vi "pyvigmentize.vi"(0 "Text Field Destination":refnum<vi>, 1 "style name (material)":string="material", 7 "String":string) -> ()   [LabVIEW 2025]
uses:
  Text Style Definition.ctl
  <vilib>/regexp/Match Regular Expression.xnode
panel:
  out "error out":errorcluster
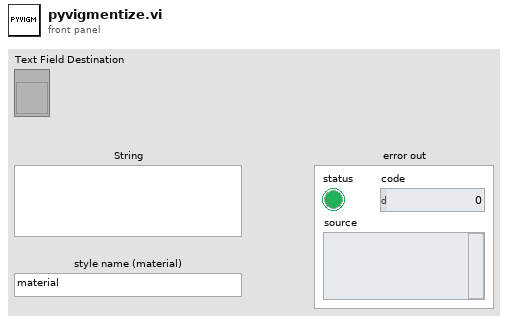
[diagram p1: front panel]
types:
  T1 = cluster{"Python version":string[], "Python version":string[]}
  T2 = typedef "Text Style Definition.ctl" = cluster{"FG color":u32, "bold":bool, "italic":bool, "underline":bool, "roman":bool, "sans":bool, "mono":bool, "strikethrough":bool, "BG color":u32}
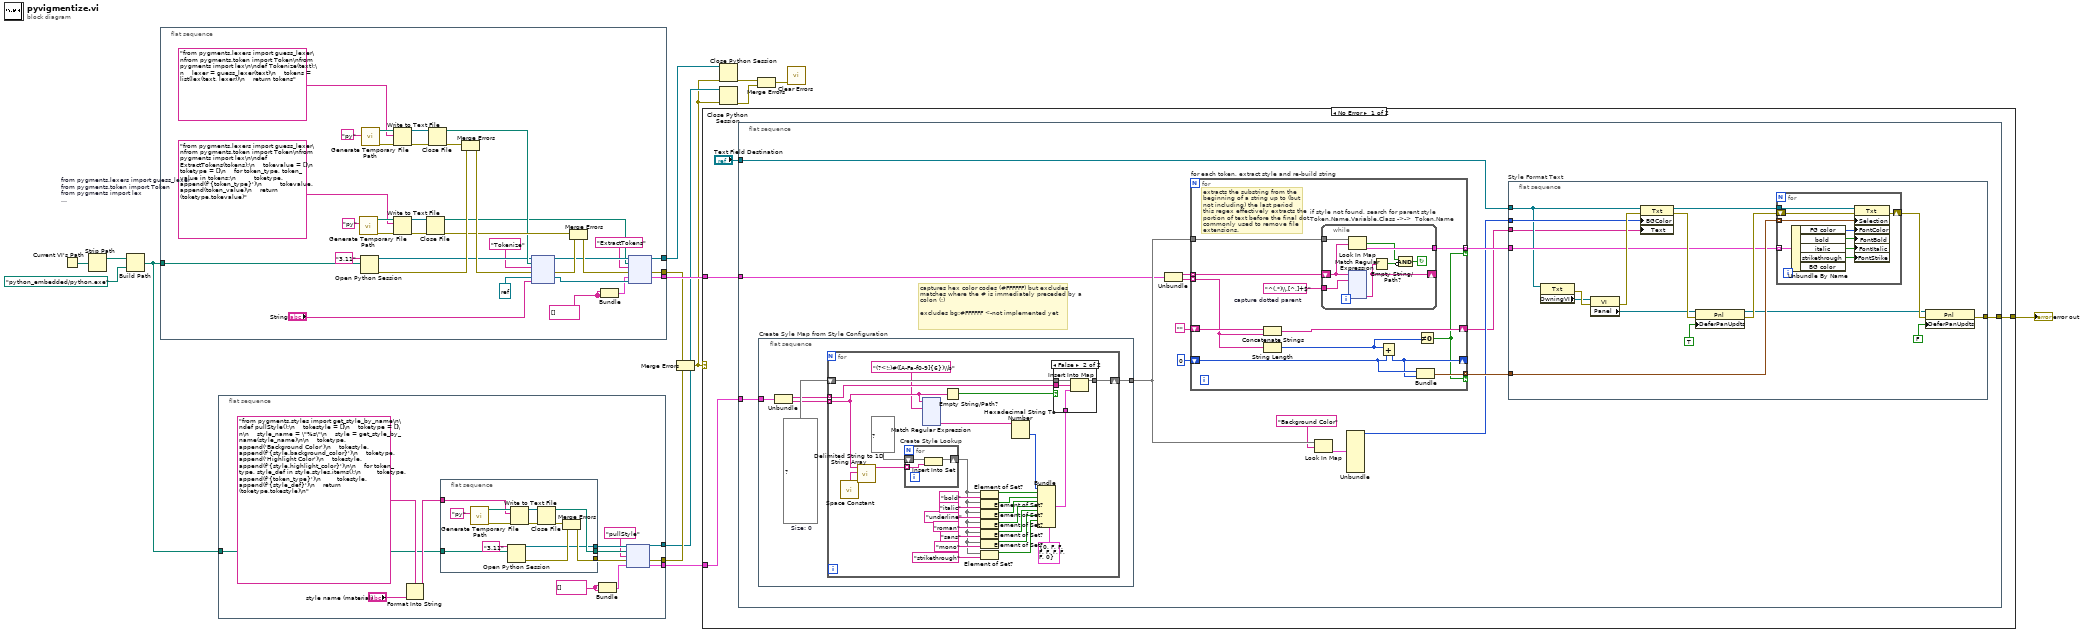
[diagram p0: block diagram]
diagram:
  n1 = Current VI's Path() -> (path=w4:path)
  n2 = Strip Path(path=w4) -> (stripped path=w2:path)  [unwired: 1 out]
  n3 = Build Path(base path=w2, name or relative path=path "python_embedded/python.exe" ("python path")) -> (appended path=w1:path)
  n4 = flat-sequence {
    tunnel: [w41] -> w12
    tunnel: [w22] -> w14
    tunnel: w1 -> [w17]
    tunnel: [w16] -> w10
    frame #0 {
      w18 = "from pygments.lexers import guess_lexer\nfrom pygments.token import Token\nfrom pygments import lex\n\ndef ExtractTokens(tokens):\n    tokevalue = []\n    toketype = []\n    for token_type, token_value in tokens:\n         toketype.append(f'{token_type}')\n         tokevalue.append(token_value)\n    return (toketype,tokevalue)"  # from pygments.lexers import guess_lexer from pygments.token import Token from pygments import lex  def ExtractTokens(tokens):     tokevalue = []     toketype = []     for token_type, token_value in tokens:          toketype.append(f'{token_type}')          tokevalue.append(token_value)     return (toketype,tokevalue)
      w19 = string[] [] ("Python version")
      n5 = call <vilib>:"Generate Temporary File Path.vi"("Temporary File Extension (tmp)"="py") -> ("error out"=w46:errorcluster, "Unique Temporary File Path"=w34:path)  [unwired: 9 in]
      n6 = Open Python Session(python version="3.11" ("Python version"), python path=w17) -> (session out=w29:refnum<k35>, error out=w44:errorcluster)  [unwired: 1 in]
      n7 = call <vilib>:"Generate Temporary File Path.vi"("Temporary File Extension (tmp)"="py") -> ("error out"=w47:errorcluster, "Unique Temporary File Path"=w35:path)  [unwired: 9 in]
      n8 = Write to Text File(file (use dialog)=w35, text="from pygments.lexers import guess_lexer\nfrom pygments.token import Token\nfrom pygments import lex\n\ndef Tokenize(text):\n    lexer = guess_lexer(text)\n    tokens = list(lex(text, lexer))\n    return tokens", error in=w47) -> (refnum out=w38:refnum<file>, error out=w48:errorcluster)  [unwired: 1 in, 1 out]
      n9 = Write to Text File(file (use dialog)=w34, text=w18, error in=w46) -> (refnum out=w32:refnum<file>, error out=w45:errorcluster)  [unwired: 1 in, 1 out]
      n10 = Close File(refnum=w32, error in=w45) -> (path=w26:path, error out=w42:errorcluster)
      n11 = Close File(refnum=w38, error in=w48) -> (path=w30:path, error out=w49:errorcluster)
      n12 = Merge Errors(w49, w44) -> (w43:errorcluster)
      n13 = node(w29, w30, "Tokenize" ("function name"), w43, refnum<k38> refnum ("Python Object Refnum"), "String") -> (w31:refnum<k35>, w40:errorcluster, w24:refnum<k38>)  [unwired: 1 in, 2 out]
      n14 = Merge Errors(w42, w40) -> (w39:errorcluster)
      n15 = Bundle("Python version"=w19, "Python version"=w19) -> (w21:T1)  [unwired: 1 in]
      n16 = node(w31, w26, "ExtractTokens" ("function name"), w39, w21, w24) -> (w16:refnum<k35>, w41:errorcluster, w22:T1)  [unwired: 1 in, 2 out]
    }
  }
  n17 = flat-sequence {
    tunnel: [w57] -> w15
    tunnel: [w52] -> w11
    tunnel: w1 -> [w51]
    tunnel: [w50] -> w9
    frame #0 {
      w56 = string[] [] ("Python version")
      n18 = Format Into String(format string="from pygments.styles import get_style_by_name\n\ndef pullStyle():\n    tokestyle = []\n    toketype = []\n\n    style_name = \"%s\"\n    style = get_style_by_name(style_name)\n\n    toketype.append('Background Color')\n    tokestyle.append(f'{style.background_color}')\n    toketype.append('Highlight Color')\n    tokestyle.append(f'{style.highlight_color}')\n\n    for token_type, style_def in style.styles.items():\n        toketype.append(f'{token_type}')\n        tokestyle.append(f'{style_def}')\n    return (toketype,tokestyle)\n" ("text"), "style name (material)") -> (resulting string=w54:string)  [unwired: 2 in, 1 out]
      n19 = flat-sequence {
        tunnel: [w66] -> w61
        tunnel: [w65] -> w60
        tunnel: [w71] -> w62
        tunnel: w54 -> [w64]
        tunnel: w51 -> [w63]
        frame #0 {
          n20 = call <vilib>:"Generate Temporary File Path.vi"("Temporary File Extension (tmp)"="py") -> ("error out"=w75:errorcluster, "Unique Temporary File Path"=w68:path)  [unwired: 9 in]
          n21 = Open Python Session(python version="3.11" ("Python version"), python path=w63) -> (session out=w65:refnum<k35>, error out=w72:errorcluster)  [unwired: 1 in]
          n22 = Write to Text File(file (use dialog)=w68, text=w64, error in=w75) -> (refnum out=w67:refnum<file>, error out=w74:errorcluster)  [unwired: 1 in, 1 out]
          n23 = Close File(refnum=w67, error in=w74) -> (path=w66:path, error out=w73:errorcluster)
          n24 = Merge Errors(w73, w72) -> (w71:errorcluster)
        }
      }
      n25 = Bundle("Python version"=w56, "Python version"=w56) -> (w58:T1)  [unwired: 1 in]
      n26 = node(w60, w61, "pullStyle" ("function name"), w62, w58) -> (w50:refnum<k35>, w52:errorcluster, w57:T1)  [unwired: 2 out]
    }
  }
  n27 = Merge Errors(w12, w11) -> (w8:errorcluster)
  n28 = case shown="No Error" w8 {
    selector: w8 -> [_ w420]
    tunnel: w15 -> [w79 _]
    tunnel: w14 -> [w78 _]
    tunnel: [w76 w420] -> w13
    frame No Error {
      n29 = flat-sequence {
        tunnel: w79 -> [w91]
        tunnel: w78 -> [w86]
        tunnel: "Text Field Destination" -> [w84]
        tunnel: [w81] -> w76
        frame #0 {
          # "captures hex color codes (#FFFFFF) but excludes matches where the # is immediately preceded by a colon (:)\n\nexcludes bg:#FFFFFF <-not implemented yet"
          n30 = flat-sequence "Create Syle Map from Style Configuration" {
            tunnel: [w125] -> w89
            tunnel: w91 -> [w123]
            frame #0 {
              w124 = map{string, T2} {}  # Size: 0
              n31 = Unbundle(w123) -> ("Python version"=w122:string[], "Python version"=w121:string[])
              n32 = for {
                tunnel: w122 -> [w134] mode=indexing
                shift-right: [w153] -> w125
                shift-left: w124 -> [w152]
                tunnel: w121 -> [w131] mode=indexing
                n33 = call <vilib>:"Space Constant.vi"() -> ("String"=w151:string)
                n34 = call <vilib>:"Delimited String to 1D String Array.vi"("delimiter"=w151, "delimited string"=w131) -> ("string array"=w132:string[])  [unwired: 9 in]
                n35 = for "Create Style Lookup" {
                  tunnel: w132 -> [w279] mode=indexing
                  shift-right: [w278] -> w127
                  shift-left: set{string} {} ("set") -> [w280]
                  n36 = Insert Into Set(10:w279, 11:w280) -> (3:w278:set{string})  [unwired: 1 out]
                }
                n37 = xnode "Match Regular Expression"("input string"=w131, "regular expression"="(?<!:)#([A-Fa-f0-9]{6})\\b") -> ("submatch 1"=w129:string)  [unwired: 4 in, 5 out]
                n38 = Empty String/Path?(string/path=w131) -> (empty?=w133:bool)
                n39 = Element of Set?(10:"bold", 11:w127) -> (3:w143:bool)
                n40 = Element of Set?(10:"italic", 11:w127) -> (3:w142:bool)
                n41 = Element of Set?(10:"underline", 11:w127) -> (3:w141:bool)
                n42 = Element of Set?(10:"roman", 11:w127) -> (3:w137:bool)
                n43 = Element of Set?(10:"sans", 11:w127) -> (3:w140:bool)
                n44 = Element of Set?(10:"mono", 11:w127) -> (3:w139:bool)
                n45 = Element of Set?(10:"strikethrough", 11:w127) -> (3:w126:bool)
                n46 = Hexadecimal String To Number(string=w129) -> (number=w150:u32)  [unwired: 2 in, 1 out]
                n47 = Bundle(cluster=T2 {"FG color"=0, "bold"=FALSE, "italic"=FALSE, "underline"=FALSE, "roman"=FALSE, "sans"=FALSE, "mono"=FALSE, "strikethrough"=FALSE, "BG color"=0}, "FG color"=w150, "bold"=w143, "italic"=w142, "underline"=w141, "roman"=w137, "sans"=w140, "mono"=w139, "strikethrough"=w126) -> (w138:T2)  [unwired: 1 in]
                n48 = case shown="False" w133 {
                  tunnel: w134 -> [_ w277]
                  tunnel: [w273 w276] -> w153
                  tunnel: w152 -> [w273 w275]
                  tunnel: w138 -> [_ w274]
                  frame True {
                  }
                  frame False {
                    n49 = Insert Into Map(map in=w275, key=w277, value=w274) -> (map out=w276:map{string, T2})  [unwired: 2 out]
                  }
                }
              }
            }
          }
          n50 = Unbundle(w86) -> ("Python version"=w83:string[], "Python version"=w82:string[])
          n51 = for "for each token, extract style and re-build string" {
            tunnel: w89 -> [w292]
            shift-right: [w286] -> _
            shift-left: 0 ("length") -> [w287]
            shift-right: [w285] -> w85
            shift-left: "" ("function name 2") -> [w291]
            tunnel: [w289] -> w92 mode=indexing if=w281
            tunnel: [w290] -> w94 mode=indexing if=w281
            tunnel: w83 -> [w284] mode=indexing
            tunnel: w82 -> [w283] mode=indexing
            w288 = "^(.*)\\.[^.]+$"  # capture dotted parent
            # "extracts the substring from the beginning of a string up to (but not including) the last period\nthis regex effectively extracts the portion of text before the final dot, commonly used to remove file extensions."
            n52 = Concatenate Strings(w291, w283) -> (w285:string)
            n53 = String Length(string=w283) -> (length=w282:i32)
            n54 = while "if style not found, search for parent style\nToken.Name.Variable.Class ->->  Token.Name" {
              tunnel: w292 -> [w300]
              tunnel: [w299] -> w290
              shift-right: [w293] -> _
              shift-left: w284 -> [w298]
              tunnel: w288 -> [w296]
              stop <- w297 continue-if-true
              n55 = Look In Map(map=w300, key=w298) -> (key not found?=w294:bool, value=w299:T2)  [unwired: 1 in]
              n56 = xnode "Match Regular Expression"("input string"=w298, "regular expression"=w296) -> ("submatch 1"=w293:string)  [unwired: 4 in, 5 out]
              n57 = Empty String/Path?(string/path=w293) -> (empty?=w295:bool)
              n58 = Compound Arithmetic op=AND(w294, invert w295) -> (w297:bool)
            }
            n59 = Add(x=w282, y=w287) -> (x+y=w286:i32)
            n60 = Bundle("length"=w287, w286) -> (w289:cluster{"length":i32, i32})  [unwired: 1 in]
            n61 = Not Equal To 0?(x=w282) -> (x != 0?=w281:bool)
          }
          n62 = Look In Map(map=w89, key="Background Color") -> (value=w90:T2)  [unwired: 1 in, 1 out]
          n63 = Unbundle(w90) -> ("FG color"=w87:u32)  [unwired: 8 out]
          n64 = flat-sequence "Style Format Text" {
            tunnel: w92 -> [w106]
            tunnel: w87 -> [w105]
            tunnel: w85 -> [w96]
            tunnel: w94 -> [w101]
            tunnel: w84 -> [w97]
            tunnel: [w95] -> w81
            frame #0 {
              n65 = property class="Txt"(reference=w97) -> (error out=w107:errorcluster, "OwningVI"=w100:refnum<vi>)  [unwired: 1 in, 1 out]
              n66 = property class="VI"(reference=w100, error in=w107) -> (error out=w109:errorcluster, "Panel"=w103:refnum<vi>)  [unwired: 1 out]
              n67 = property class="Txt"(reference=w97, error in=w109, "BGColor"=w105, "Text"=w96) -> (reference out=w102:refnum<vi>, error out=w108:errorcluster)
              n68 = property class="Pnl"(reference=w103, error in=w108, "DeferPanUpdts"=TRUE ("Defer Panel Updates")) -> (reference out=w104:refnum<vi>, error out=w111:errorcluster)
              n69 = for {
                tunnel: w102 -> [w119]
                tunnel: w106 -> [w118] mode=indexing
                tunnel: w101 -> [w117] mode=indexing
                shift-right: [w120] -> w110
                shift-left: w111 -> [w114]
                n70 = Unbundle By Name(w117) -> ("FG color"=w116:u32, "bold"=w113:bool, "italic"=w112:bool, "strikethrough"=w115:bool)  [unwired: 1 out]
                n71 = property class="Txt"(reference=w119, error in=w114, "Selection"=w118, "FontColor"=w116, "FontBold"=w113, "FontItalic"=w112, "FontStrike"=w115) -> (error out=w120:errorcluster)  [unwired: 1 out]
              }
              n72 = property class="Pnl"(reference=w104, error in=w110, "DeferPanUpdts"=FALSE ("Defer Panel Updates")) -> (error out=w95:errorcluster)  [unwired: 1 out]
            }
          }
        }
      }
    }
    frame Error {
    }
  }
  "error out" <- w13
  n73 = Close Python Session(session in=w10, error in=w8) -> (11:w7:errorcluster)
  n74 = Close Python Session(session in=w9, error in=w8) -> (11:w6:errorcluster)
  n75 = Merge Errors(w7, w6) -> (w5:errorcluster)
  n76 = call <vilib>:"Clear Errors.vi"("error in (no error)"=w5) -> ()  [unwired: 5 in, 2 out]
